vi "wait Targets match.vi"(10 "status":T2, 11 "Mercury Targets":T1) -> (1 "Target AND Rate Match":bool, 2 "Target ~ Magnet":bool, 3 "Target ~ PS":bool)   [LabVIEW 2016, in "Mercury-1820-API.lvlib"]
uses:
  Mercury-1820-API.lvlib
  Typedefs/Status.ctl
  Typedefs/Targets.ctl
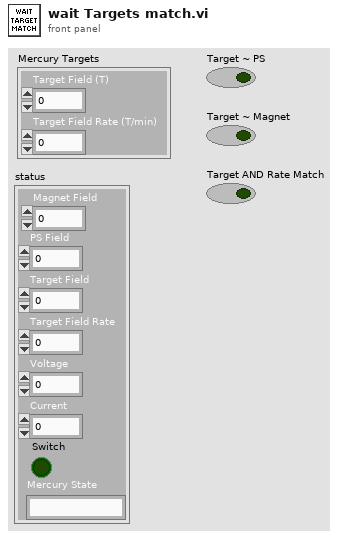
[diagram p1: front panel]
types:
  T1 = typedef "Mercury-1820-API.lvlib/Targets.ctl" = cluster{"Target Field (T)":dbl, "Target Field Rate (T/min)":dbl}
  T2 = typedef "Mercury-1820-API.lvlib/Status.ctl" = cluster{"Magnet Field":dbl, "PS Field":dbl, "Target Field":dbl, "Target Field Rate":dbl, "Voltage":dbl, "Current":dbl, "Switch":bool, "Mercury State":string}
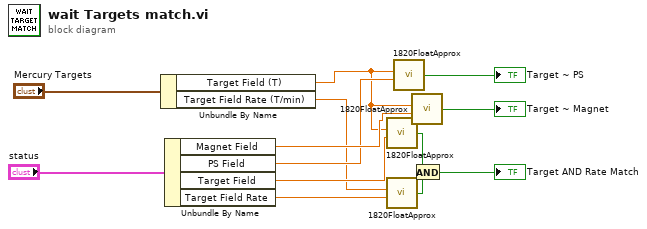
[diagram p0: block diagram]
diagram:
  n1 = Unbundle By Name("Mercury Targets") -> ("Target Field (T)"=w2:dbl, "Target Field Rate (T/min)"=w9:dbl)
  n2 = Unbundle By Name("status") -> ("Magnet Field"=w12:dbl, "PS Field"=w11:dbl, "Target Field"=w10:dbl, "Target Field Rate"=w7:dbl)
  n3 = call "1820FloatApprox.vi"("y"=w10, "x"=w2) -> ("x ~ y?"=w6:bool)  [unwired: 2 in]
  n4 = call "1820FloatApprox.vi"("y"=w7, "x"=w9) -> ("x ~ y?"=w8:bool)  [unwired: 2 in]
  n5 = call "1820FloatApprox.vi"("y"=w11, "x"=w2) -> ("x ~ y?"=→"Target ~ PS":bool)  [unwired: 2 in]
  n6 = call "1820FloatApprox.vi"("y"=w12, "x"=w2) -> ("x ~ y?"=→"Target ~ Magnet":bool)  [unwired: 2 in]
  n7 = And(x=w6, y=w8) -> (x .and. y?=→"Target AND Rate Match":bool)
